vi "Tester.vi"() -> ()   [LabVIEW 2016]
uses:
  IMessageTransport/IMessageTransport.lvclass
  QueueMessageTransport/QueueMessageTransport.lvclass
  C:/Users/Dzak/Desktop/TD[S]CC/Classes/Message Transport/IMessageTransport/IMessageTransport.lvclass
  QMHMessagePayload/QMHMessagePayload.lvclass
  C:/Users/Dzak/Desktop/TD[S]CC/Classes/Message Transport/IMessagePayload/IMessagePayload.lvclass
  NotifierMessageTransport/NotifierMessageTransport.lvclass
  IMessagePayload/IMessagePayload.lvclass
  UserEventMessageTransport/UserEventMessageTransport.lvclass
panel:
  out "Array":cluster{"State":enum16{""}, "Data":variant}[](array[cluster])
  in  "State":enum16{""}(ring)
  out "IMessageTransport out":refnum<class "IMessageTransport.lvclass">
  out "error out":errorcluster
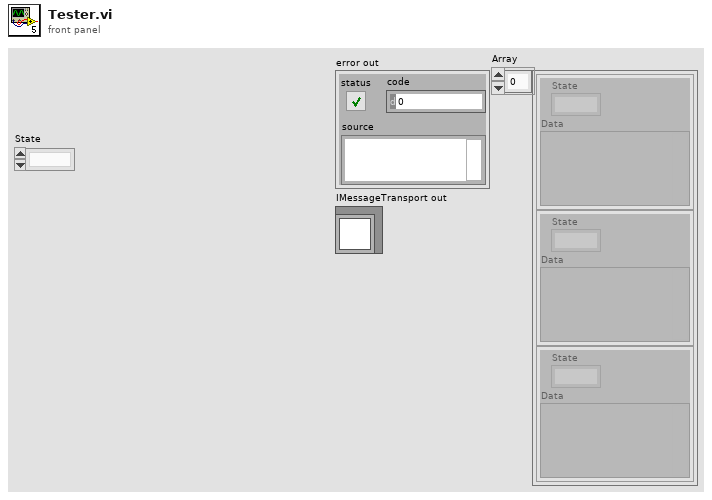
[diagram p1: front panel]
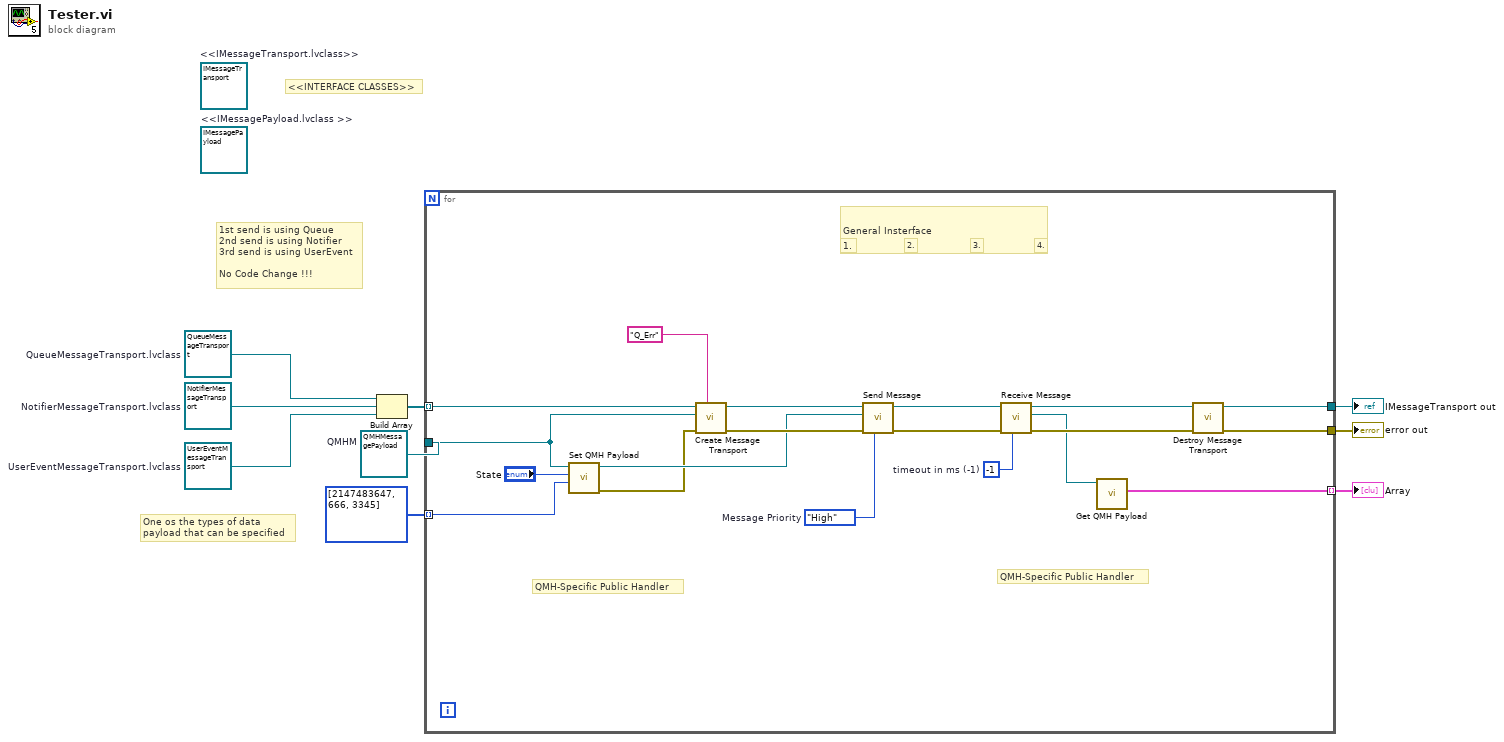
[diagram p0: block diagram]
diagram:
  w1 = refnum<class "UserEventMessageTransport.lvclass"> refnum  # UserEventMessageTransport.lvclass
  (unwired) refnum<class "IMessagePayload.lvclass"> refnum  # <<IMessagePayload.lvclass >>
  w4 = refnum<class "NotifierMessageTransport.lvclass"> refnum  # NotifierMessageTransport.lvclass
  (unwired) refnum<class "IMessageTransport.lvclass"> refnum  # <<IMessageTransport.lvclass>>
  w7 = refnum<class "QMHMessagePayload.lvclass"> refnum  # QMHM
  w5 = refnum<class "QueueMessageTransport.lvclass"> refnum  # QueueMessageTransport.lvclass
  # "<<INTERFACE CLASSES>>"
  # "One os the types of data\npayload that can be specified"
  # "1st send is using Queue\n2nd send is using Notifier\n3rd send is using UserEvent\n\nNo Code Change !!!"
  n1 = Build Array(w5, w4, w1) -> (w3:refnum<class "IMessageTransport.lvclass">[])
  n2 = for {
    tunnel: [w28] -> w9
    tunnel: w7 -> [w16]
    tunnel: [w14] -> w6 mode=indexing
    tunnel: w3 -> [w10] mode=indexing
    tunnel: [w27] -> w8
    tunnel: i32[] [2147483647, 666, 3345] -> [w11] mode=indexing
    w20 = -1  # timeout in ms (-1)
    w24 = enum16{"Normal", "High"}."High"  # Message Priority
    # "QMH-Specific Public Handler"
    # "QMH-Specific Public Handler"
    # "4."
    # "3."
    # "2."
    # "1."
    # "General Insterface"
    n3 = call "Set QMH Payload.vi"("Data"=w11, "State"="State", "IMessagePayload in"=w16) -> ("error out"=w13:errorcluster, "IMessagePayload"=w18:refnum<class "IMessagePayload.lvclass">)  [unwired: 7 in]
    n4 = call-dynamic "Create Message Transport.vi"("Transport Name"="Q_Err" ("Q Name"), "error in"=w13, "Transport Payload type"=w16, "IMessageTransport in"=w10) -> ("error out"=w25:errorcluster, "IMessageTransport out"=w23:refnum<class "IMessageTransport.lvclass">)  [unwired: 6 in]
    n5 = call-dynamic "Send Message.vi"("Message Priority"=w24, "error in"=w25, "Message Payload in"=w18, "IMessageTransport in"=w23) -> ("error out"=w22:errorcluster, "IMessageTransport out"=w15:refnum<class "IMessageTransport.lvclass">)  [unwired: 6 in]
    n6 = call-dynamic "Receive Message.vi"("timeout in ms (-1)"=w20, "error in"=w22, "IMessageTransport in"=w15) -> ("error out"=w19:errorcluster, "Q Element"=w17:refnum<class "IMessagePayload.lvclass">, "IMessageTransport out"=w21:refnum<class "IMessageTransport.lvclass">)  [unwired: 6 in]
    n7 = call "Get QMH Payload.vi"("IMessagePayload in"=w17) -> ("QMH Payload"=w14:cluster{"State":enum16{""}, "Data":variant})  [unwired: 8 in, 2 out]
    n8 = call-dynamic "Destroy Message Transport.vi"("error in"=w19, "IMessageTransport in"=w21) -> ("error out"=w28:errorcluster, "IMessageTransport out"=w27:refnum<class "IMessageTransport.lvclass">)  [unwired: 8 in]
  }
  "error out" <- w9
  "IMessageTransport out" <- w8
  "Array" <- w6
